vi "Create Spectra Figure 2.0.vi"() -> ()   [LabVIEW 2021]
uses:
  <vilib>/Heliosphere Research LLC/Advanced Plotting Toolkit/api_annotations/LabelProperties.ctl
  <vilib>/Heliosphere Research LLC/Advanced Plotting Toolkit/properties/Text.ctl
  <vilib>/Heliosphere Research LLC/Advanced Plotting Toolkit/typedefs/PlotColor.ctl
  <vilib>/Heliosphere Research LLC/Advanced Plotting Toolkit/properties/Text_FontSize.ctl
  <vilib>/Heliosphere Research LLC/Advanced Plotting Toolkit/properties/Text_FontStyle.ctl
  <vilib>/Heliosphere Research LLC/Advanced Plotting Toolkit/api_figure/TicksProperties.ctl
  <vilib>/Heliosphere Research LLC/Advanced Plotting Toolkit/api_plotting/LineProperties.ctl
  <vilib>/Heliosphere Research LLC/Advanced Plotting Toolkit/properties/Line.ctl
  <vilib>/Heliosphere Research LLC/Advanced Plotting Toolkit/properties/Line_Style.ctl
  <vilib>/Heliosphere Research LLC/Advanced Plotting Toolkit/properties/Marker.ctl
  <vilib>/Heliosphere Research LLC/Advanced Plotting Toolkit/properties/Marker_Style.ctl
  <vilib>/Heliosphere Research LLC/Advanced Plotting Toolkit/properties/Display.ctl
  <vilib>/regexp/Match Regular Expression.xnode
  <vilib>/Heliosphere Research LLC/Advanced Plotting Toolkit/Advanced Plotting Toolkit.lvlib
  <vilib>/Analysis/NI_AALPro.lvlib
panel:
  out "Pressure":picture
  out "Speed Profiles":picture
  out "Full Spectrum":picture
  out "Trimmed Spectra":picture
  out "Bar Plot":picture
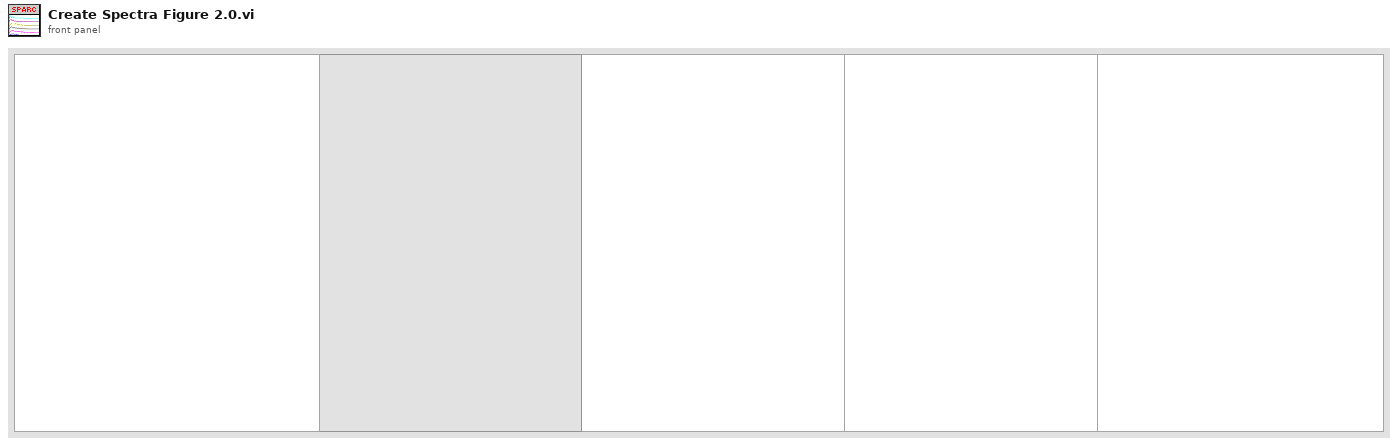
[diagram p1: front panel]
types:
  T1 = typedef "Advanced Plotting Toolkit.lvlib/LineProperties.ctl" = cluster{"Line":T2, "Marker":T5, "Display":T7}
  T2 = typedef "Advanced Plotting Toolkit.lvlib/Line.ctl" = cluster{"Style":T3, "Color":T4, "Width":sgl}
  T3 = typedef "Advanced Plotting Toolkit.lvlib/Line_Style.ctl" = enum16{"Automatic", "Solid", "Dashed", "Dotted", "Dash-dot", "Invisible"}
  T4 = typedef "Advanced Plotting Toolkit.lvlib/PlotColor.ctl" = u32
  T5 = typedef "Advanced Plotting Toolkit.lvlib/Marker.ctl" = cluster{"Style":T6, "Color":T4, "Size":dbl}
  T6 = typedef "Advanced Plotting Toolkit.lvlib/Marker_Style.ctl" = enum16{"Automatic", "Circle", "Square", "Triangle", "Diamond", "Star", "Invisible"}
  T7 = typedef "Advanced Plotting Toolkit.lvlib/Display.ctl" = cluster{"Alpha":dbl, "Z Order":dbl}
  T8 = typedef "Advanced Plotting Toolkit.lvlib/TicksProperties.ctl" = cluster{"Text":T9}
  T9 = typedef "Advanced Plotting Toolkit.lvlib/Text.ctl" = cluster{"Color":T4, "Background Color":T4, "Font Size (points)":T10, "Font Style":T11, "Rotation Angle":dbl}
  T10 = typedef "Advanced Plotting Toolkit.lvlib/Text_FontSize.ctl" = i32
  T11 = typedef "Advanced Plotting Toolkit.lvlib/Text_FontStyle.ctl" = enum16{"Automatic", "Normal", "Italic", "Bold"}
  T12 = typedef "Advanced Plotting Toolkit.lvlib/LabelProperties.ctl" = cluster{"Text":T9}
  T13 = typedef "Advanced Plotting Toolkit.lvlib/PlotID.ctl" = i32
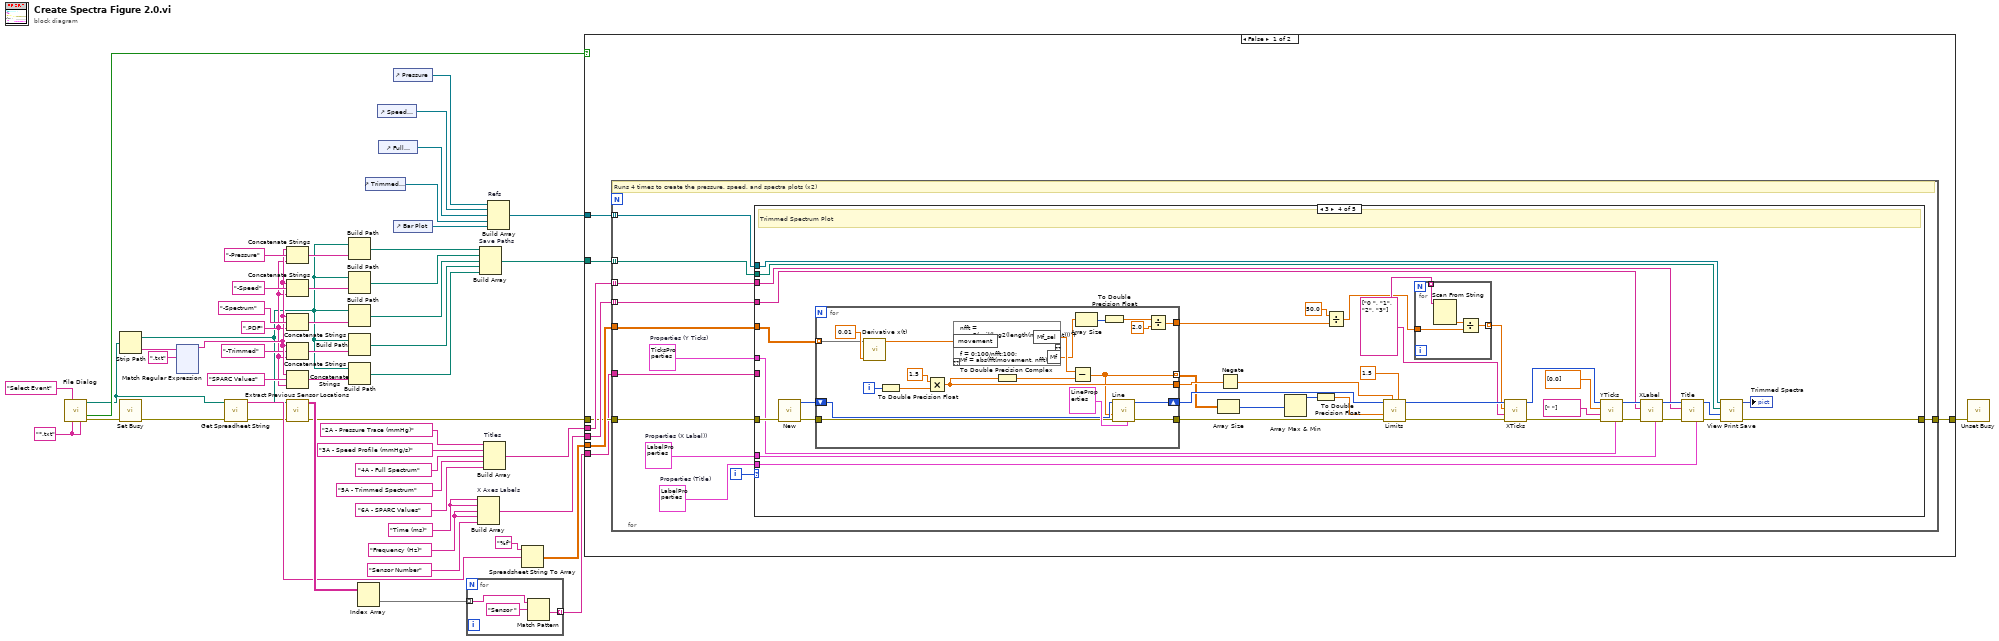
[diagram p0: block diagram]
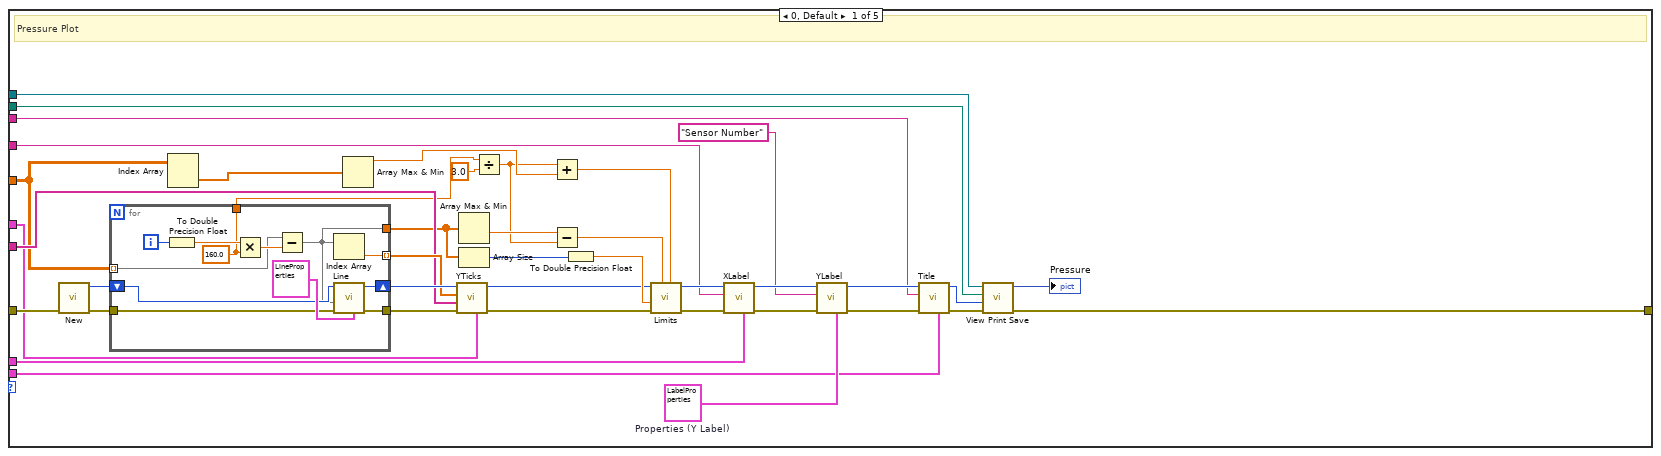
[diagram p2: hidden frame]
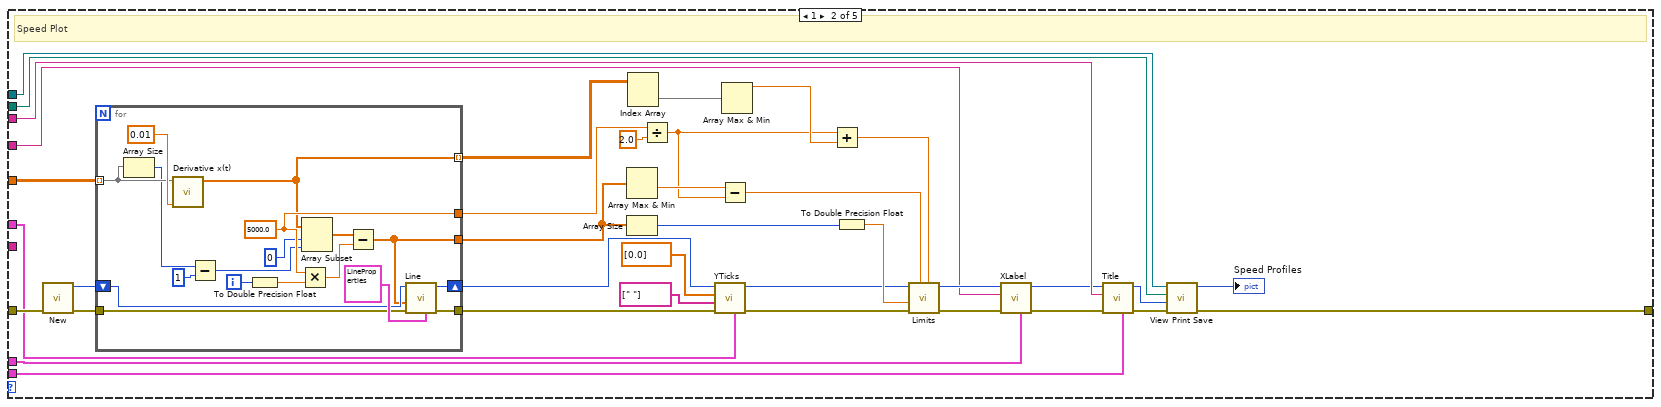
[diagram p3: hidden frame]
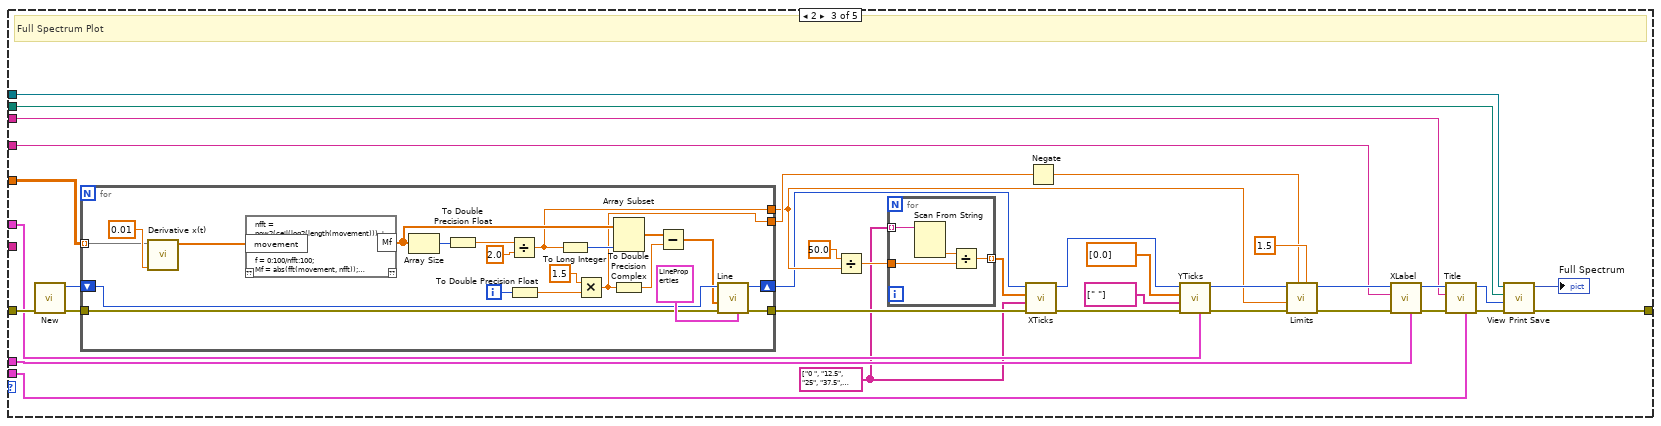
[diagram p4: hidden frame]
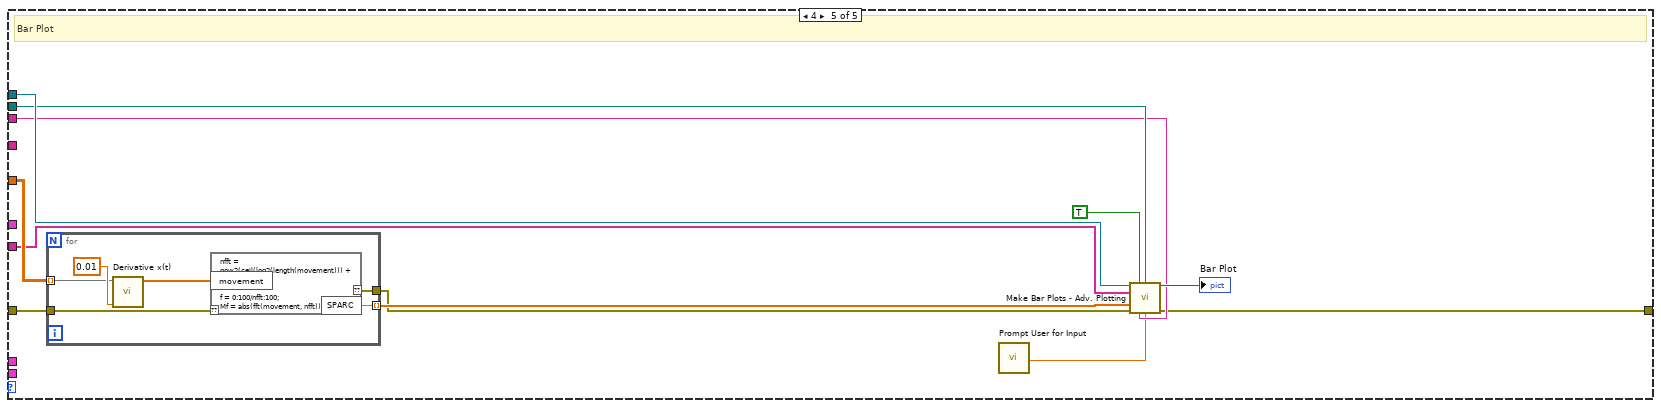
[diagram p5: hidden frame]
diagram:
  w20 = ".PDF" ("string")
  w38 = "Frequency (Hz)" ("Label")
  w39 = "Time (ms)" ("Label")
  w49 = "*.txt" ("pattern label")
  n1 = call "File Dialog"("prompt"="Select Event", "pattern (all files)"=w49, "pattern label"=w49) -> ("selected path"=w26:path, "cancelled"=w51:bool, "error out"=w45:errorcluster)  [unwired: 9 in, 1 out]
  n2 = Strip Path(path=w26) -> (stripped path=w4:path, name=w35:string)
  n3 = call <vilib>:"Set Busy.vi"("error in (no error)"=w45) -> ("error out"=w3:errorcluster)  [unwired: 9 in, 1 out]
  n4 = xnode "Match Regular Expression"("input string"=w35, "regular expression"=".txt") -> ("before match"=w25:string)  [unwired: 4 in, 4 out]
  n5 = call "Get Spreadheet String.vi"("error in (no error)"=w3, "File Path"=w26) -> ("error out"=w2:errorcluster, "Spreadsheet String"=w46:string)  [unwired: 8 in]
  n6 = Concatenate Strings(w25, "-Pressure" ("string"), w20) -> (w37:string)
  n7 = Concatenate Strings(w25, "-Speed" ("string"), w20) -> (w30:string)
  n8 = Concatenate Strings(w25, "-Spectrum" ("string"), w20) -> (w31:string)
  n9 = Concatenate Strings(w25, "-Trimmed" ("string"), w20) -> (w22:string)
  n10 = Concatenate Strings(w25, "SPARC Values" ("string"), w20) -> (w32:string)
  n11 = call "Extract Previous Sensor Locations.vi"("error in (no error)"=w2, "Folder Path"=w4) -> ("error out"=w1:errorcluster, "Sensors"=w47:string[][])  [unwired: 7 in, 1 out]
  n12 = Build Path(base path=w4, name or relative path=w37) -> (appended path=w33:path)
  n13 = Build Path(base path=w4, name or relative path=w30) -> (appended path=w24:path)
  n14 = Build Path(base path=w4, name or relative path=w31) -> (appended path=w23:path)
  n15 = Build Path(base path=w4, name or relative path=w22) -> (appended path=w19:path)
  n16 = Build Path(base path=w4, name or relative path=w32) -> (appended path=w8:path)
  n17 = Index Array(array=w47) -> (element=w44:string[])  [unwired: 2 in]
  n18 = control-ref of="Trimmed Spectra"() -> (w12:refnum<vi>)
  n19 = control-ref of="Speed Profiles"() -> (w14:refnum<vi>)
  n20 = control-ref of="Full Spectrum"() -> (w13:refnum<vi>)
  n21 = control-ref of="Pressure"() -> (w15:refnum<vi>)
  n22 = control-ref of="Bar Plot"() -> (w9:refnum<vi>)
  n23 = for {
    tunnel: w44 -> [w55] mode=indexing
    tunnel: [w53] -> w7 mode=indexing
    n24 = Match Pattern(string=w55, regular expression="Sensor ") -> (after substring=w53:string)  [unwired: 1 in, 3 out]
  }
  n25 = Build Array "X Axes Labels"(w39, w39, w38, w38, "Sensor Number" ("Label")) -> (w16:string[])
  n26 = Build Array "Save Paths"(w33, w24, w23, w19, w8) -> (w17:path[])
  n27 = Build Array "Titles"("2A - Pressure Trace (mmHg)" ("Title"), "3A - Speed Profile (mmHg/s)" ("Title"), "4A - Full Spectrum" ("Title"), "5A - Trimmed Spectrum" ("Title"), "6A - SPARC Values" ("Title")) -> (w18:string[])
  n28 = Build Array "Refs"(w15, w14, w13, w12, w9) -> (w11:refnum<vi>[])
  n29 = Spreadsheet String To Array(format string="%f", spreadsheet string=w46) -> (array=w48:dbl[][])  [unwired: 2 in]
  n30 = case shown="False" w51 {
    tunnel: w1 -> [w58 w324]
    tunnel: w48 -> [w61 _]
    tunnel: w18 -> [w63 _]
    tunnel: w17 -> [w59 _]
    tunnel: w16 -> [w62 _]
    tunnel: w11 -> [w60 _]
    tunnel: [w57 w324] -> w10
    tunnel: w7 -> [w56 _]
    frame False {
      n31 = for {
        tunnel: w63 -> [w69] mode=indexing
        tunnel: w62 -> [w65] mode=indexing
        tunnel: w61 -> [w72]
        tunnel: w60 -> [w73] mode=indexing
        tunnel: w59 -> [w74] mode=indexing
        tunnel: w58 -> [w71]
        tunnel: [w70] -> w57
        tunnel: w56 -> [w68]
        i -> [w75]
        w64 = T8 {"Text"={"Color"=2147483647, "Background Color"=2147483647, "Font Size (points)"=-3, "Font Style"=enum."Bold", "Rotation Angle"=0.0}}  # Properties (Y Ticks)
        w66 = T12 {"Text"={"Color"=2147483647, "Background Color"=2147483647, "Font Size (points)"=-3, "Font Style"=enum."Bold", "Rotation Angle"=nan}}  # Properties (X Label))
        w67 = T12 {"Text"={"Color"=2147483647, "Background Color"=2147483647, "Font Size (points)"=-4, "Font Style"=enum."Bold", "Rotation Angle"=nan}}  # Properties (Title)
        # "Runs 4 times to create the pressure, speed, and spectra plots (x2)"
        n32 = case shown="3" w75 {
          tunnel: w74 -> [w115 w163 w216 w279 w312]
          tunnel: w73 -> [w114 w164 w217 w280 w313]
          tunnel: w72 -> [w81 w148 w196 w276 w315]
          tunnel: w71 -> [w110 w158 w212 w275 w307]
          tunnel: [w109 w161 w211 w274 w309] -> w70
          tunnel: w69 -> [w103 w139 w200 w265 w311]
          tunnel: w68 -> [w88 _ _ _ w310]
          tunnel: w67 -> [w102 w142 w195 w264 _]
          tunnel: w66 -> [w76 w138 w198 w262 _]
          tunnel: w65 -> [w95 w143 w199 w263 _]
          tunnel: w64 -> [w77 w130 w197 w261 _]
          frame 0, Default {
            w106 = T12 {"Text"={"Color"=2147483647, "Background Color"=2147483647, "Font Size (points)"=-3, "Font Style"=enum."Bold", "Rotation Angle"=nan}}  # Properties (Y Label)
            # "Pressure Plot"
            n33 = call <vilib>:"New.vi"("error in (no error)"=w110) -> ("error out"=w112:errorcluster, "Plot ID"=w111:T13)  [unwired: 9 in]
            n34 = for {
              tunnel: w81 -> [w119] mode=indexing
              shift-right: [w126] -> w90
              shift-left: w111 -> [w125]
              tunnel: w112 -> [w124]
              tunnel: [w123] -> w93
              tunnel: [w118] -> w84
              tunnel: [w117] -> w89 mode=indexing
              tunnel: [w116] -> w80
              i -> [w122]
              w116 = 160.0 ("y")
              n35 = To Double Precision Float(number=w122) -> (double precision float=w121:dbl)
              n36 = Multiply(x=w121, y=w116) -> (x*y=w120:dbl)
              n37 = Subtract(x=w119, y=w120) -> (x-y=w118:dbl[])
              n38 = Index Array(array=w118) -> (element=w117:dbl)  [unwired: 1 in]
              n39 = call <vilib>:"Line.vi"("Properties"=T1 {"Line"={"Style"=enum."Automatic", "Color"=2147483647, "Width"=2.0}, "Marker"={"Style"=enum."Automatic", "Color"=2147483647, "Size"=nan}, "Display"={"Alpha"=nan, "Z Order"=nan}}, "error in (no error)"=w124, "Y Data"=w118, "Plot ID"=w125) -> ("error out"=w123:errorcluster, "Plot ID out"=w126:T13)  [unwired: 6 in]
            }
            n40 = Index Array(array=w81) -> (element=w87:dbl[])  [unwired: 2 in]
            n41 = Array Max & Min(array=w87) -> (max value=w86:dbl)  [unwired: 3 out]
            n42 = call <vilib>:"YTicks.vi"("Properties"=w77, "error in (no error)"=w93, "Tick Labels"=w88, "Tick Locations"=w89, "Plot ID"=w90) -> ("error out"=w92:errorcluster, "Plot ID Out"=w91:T13)  [unwired: 5 in]
            n43 = Array Max & Min(array=w84) -> (min value=w83:dbl)  [unwired: 3 out]
            n44 = Array Size(array=w84) -> (size(s)=w97:i32)
            n45 = Divide(x=w80, y=3.0) -> (x/y=w78:dbl)
            n46 = Add(x=w78, y=w86) -> (x+y=w85:dbl)
            n47 = Subtract(x=w83, y=w78) -> (x-y=w82:dbl)
            n48 = To Double Precision Float(number=w97) -> (double precision float=w96:dbl)
            n49 = call <vilib>:"Limits.vi"("Y Max"=w85, "Y Min"=w82, "error in (no error)"=w92, "X Max"=w96, "Plot ID"=w91) -> ("error out"=w100:errorcluster, "Plot ID Out"=w99:T13)  [unwired: 5 in]
            n50 = call <vilib>:"XLabel.vi"("Properties"=w76, "error in (no error)"=w100, "Label"=w95, "Plot ID"=w99) -> ("error out"=w101:errorcluster, "Plot ID out"=w98:T13)  [unwired: 6 in]
            n51 = call <vilib>:"YLabel.vi"("Properties"=w106, "error in (no error)"=w101, "Label"="Sensor Number", "Plot ID"=w98) -> ("error out"=w107:errorcluster, "Plot ID out"=w108:T13)  [unwired: 6 in]
            n52 = call <vilib>:"Title.vi"("Properties"=w102, "error in (no error)"=w107, "Title"=w103, "Plot ID"=w108) -> ("error out"=w104:errorcluster, "Plot ID out"=w105:T13)  [unwired: 6 in]
            n53 = call "View Print Save.vi"("error in (no error)"=w104, "Plot ID in"=w105, "appended path"=w115, "Picture in"=w114) -> ("error out"=w109:errorcluster, "Picture"=→"Pressure":picture)  [unwired: 6 in]
          }
          frame 1 {
            # "Speed Plot"
            n54 = call <vilib>:"New.vi"("error in (no error)"=w158) -> ("error out"=w160:errorcluster, "Plot ID"=w159:T13)  [unwired: 9 in]
            n55 = for {
              tunnel: w148 -> [w171] mode=indexing
              shift-right: [w181] -> w141
              shift-left: w159 -> [w180]
              tunnel: w160 -> [w179]
              tunnel: [w178] -> w145
              tunnel: [w173] -> w146
              tunnel: [w172] -> w134
              tunnel: [w165] -> w129 mode=indexing
              i -> [w176]
              w172 = 5000.0 ("x")
              n56 = Array Size(array=w171) -> (size(s)=w170:i32)
              n57 = call <vilib>:"Derivative x(t).vi"("dt"=0.01, "X"=w171) -> ("dX/dt"=w165:dbl[])  [unwired: 8 in, 1 out]
              n58 = Subtract(x=w170, y=1) -> (x-y=w168:i32)
              n59 = To Double Precision Float(number=w176) -> (double precision float=w175:dbl)
              n60 = Multiply(x=w172, y=w175) -> (x*y=w174:dbl)
              n61 = Array Subset(array=w165, index=0, length=w168) -> (w166:dbl[])
              n62 = Subtract(x=w166, y=w174) -> (x-y=w173:dbl[])
              n63 = call <vilib>:"Line.vi"("Properties"=T1 {"Line"={"Style"=enum."Automatic", "Color"=2147483647, "Width"=2.0}, "Marker"={"Style"=enum."Automatic", "Color"=2147483647, "Size"=nan}, "Display"={"Alpha"=nan, "Z Order"=nan}}, "error in (no error)"=w179, "Y Data"=w173, "Plot ID"=w180) -> ("error out"=w178:errorcluster, "Plot ID out"=w181:T13)  [unwired: 6 in]
            }
            n64 = Array Max & Min(array=w146) -> (min value=w150:dbl)  [unwired: 3 out]
            n65 = Array Size(array=w146) -> (size(s)=w155:i32)
            n66 = Index Array(array=w129) -> (element=w128:dbl[])  [unwired: 2 in]
            n67 = Divide(x=w134, y=2.0) -> (x/y=w135:dbl)
            n68 = call <vilib>:"YTicks.vi"("Properties"=w130, "error in (no error)"=w145, "Tick Labels"=string[] [" "], "Tick Locations"=dbl[] [0.0], "Plot ID"=w141) -> ("error out"=w153:errorcluster, "Plot ID Out"=w152:T13)  [unwired: 5 in]
            n69 = Subtract(x=w150, y=w135) -> (x-y=w149:dbl)
            n70 = Array Max & Min(array=w128) -> (max value=w147:dbl)  [unwired: 3 out]
            n71 = Add(x=w135, y=w147) -> (x+y=w151:dbl)
            n72 = To Double Precision Float(number=w155) -> (double precision float=w154:dbl)
            n73 = call <vilib>:"Limits.vi"("Y Max"=w151, "Y Min"=w149, "error in (no error)"=w153, "X Max"=w154, "Plot ID"=w152) -> ("error out"=w157:errorcluster, "Plot ID Out"=w156:T13)  [unwired: 5 in]
            n74 = call <vilib>:"XLabel.vi"("Properties"=w138, "error in (no error)"=w157, "Label"=w143, "Plot ID"=w156) -> ("error out"=w132:errorcluster, "Plot ID out"=w131:T13)  [unwired: 6 in]
            n75 = call <vilib>:"Title.vi"("Properties"=w142, "error in (no error)"=w132, "Title"=w139, "Plot ID"=w131) -> ("error out"=w144:errorcluster, "Plot ID out"=w140:T13)  [unwired: 6 in]
            n76 = call "View Print Save.vi"("error in (no error)"=w144, "Plot ID in"=w140, "appended path"=w163, "Picture in"=w164) -> ("error out"=w161:errorcluster, "Picture"=→"Speed Profiles":picture)  [unwired: 6 in]
          }
          frame 2 {
            w184 = string[] ["0 ", "12.5", "25", "37.5", "50"] ("Tick Labels")
            # "Full Spectrum Plot"
            n77 = call <vilib>:"New.vi"("error in (no error)"=w212) -> ("error out"=w214:errorcluster, "Plot ID"=w213:T13)  [unwired: 9 in]
            n78 = for {
              tunnel: w196 -> [w235] mode=indexing
              shift-right: [w241] -> w187
              shift-left: w213 -> [w240]
              tunnel: w214 -> [w239]
              tunnel: [w238] -> w186
              tunnel: [w226] -> w191
              tunnel: [w222] -> w193
              i -> [w230]
              n79 = call <vilib>:"Derivative x(t).vi"("dt"=0.01, "X"=w235) -> ("dX/dt"=w236:dbl[])  [unwired: 8 in, 1 out]
              n80 = script code="nfft = pow2(ceil(log2(length(movement))) + 4);\n\nf = 0:100/nfft:100;\nMf = abs(fft(movement, nfft));\nMf = Mf/max(Mf);\n\nfc_inx = find(f<=3);\nf_sel = f(fc_inx);\nMf_sel = Mf(fc_inx);\n\n\ninx = find((Mf_sel>=0.01));\nfc_inx = inx(1):inx(end);\nf_sel = f_sel(fc_inx);\nMf_sel = Mf_sel(fc_inx);\n\nSPARC = -sum(sqrt((diff(f_sel)/f_sel(end)-f_sel(1)).^2+(diff(Mf_sel).^2)));"("movement"=w236) -> ("Mf"=w229:cdb[])  [unwired: 1 in, 1 out]
              n81 = Array Size(array=w229) -> (size(s)=w234:i32)
              n82 = To Double Precision Float(number=w234) -> (double precision float=w233:dbl)
              n83 = Divide(x=w233, y=2.0) -> (x/y=w226:dbl)
              n84 = To Double Precision Float(number=w230) -> (double precision float=w231:dbl)
              n85 = To Long Integer(number=w226) -> (32bit integer=w228:i32)
              n86 = Multiply(x=1.5, y=w231) -> (x*y=w222:dbl)
              n87 = Array Subset(array=w229, length=w228) -> (w223:cdb[])  [unwired: 1 in]
              n88 = To Double Precision Complex(1:w222) -> (0:w227:cdb)
              n89 = Subtract(x=w223, y=w227) -> (x-y=w224:cdb[])
              n90 = call <vilib>:"Line.vi"("Properties"=T1 {"Line"={"Style"=enum."Automatic", "Color"=2147483647, "Width"=2.0}, "Marker"={"Style"=enum."Automatic", "Color"=2147483647, "Size"=nan}, "Display"={"Alpha"=nan, "Z Order"=nan}}, "error in (no error)"=w239, "Y Data"=w224, "Plot ID"=w240) -> ("error out"=w238:errorcluster, "Plot ID out"=w241:T13)  [unwired: 6 in]
            }
            n91 = Divide(x=50.0, y=w191) -> (x/y=w185:dbl)
            n92 = for {
              tunnel: w184 -> [w221] mode=indexing
              tunnel: w185 -> [w219]
              tunnel: [w218] -> w183 mode=indexing
              n93 = Scan From String(input string=w221) -> (output 1=w220:dbl)  [unwired: 4 in, 3 out]
              n94 = Divide(x=w220, y=w219) -> (x/y=w218:dbl)
            }
            n95 = call <vilib>:"XTicks.vi"("error in (no error)"=w186, "Tick Labels"=w184, "Tick Locations"=w183, "Plot ID"=w187) -> ("error out"=w189:errorcluster, "Plot ID Out"=w188:T13)  [unwired: 6 in]
            n96 = Negate(x=w193) -> (-x=w192:dbl)
            n97 = call <vilib>:"YTicks.vi"("Properties"=w197, "error in (no error)"=w189, "Tick Labels"=string[] [" "], "Tick Locations"=dbl[] [0.0], "Plot ID"=w188) -> ("error out"=w208:errorcluster, "Plot ID Out"=w207:T13)  [unwired: 5 in]
            n98 = call <vilib>:"Limits.vi"("Y Max"=1.5, "Y Min"=w192, "error in (no error)"=w208, "X Max"=w191, "Plot ID"=w207) -> ("error out"=w210:errorcluster, "Plot ID Out"=w209:T13)  [unwired: 5 in]
            n99 = call <vilib>:"XLabel.vi"("Properties"=w198, "error in (no error)"=w210, "Label"=w199, "Plot ID"=w209) -> ("error out"=w204:errorcluster, "Plot ID out"=w203:T13)  [unwired: 6 in]
            n100 = call <vilib>:"Title.vi"("Properties"=w195, "error in (no error)"=w204, "Title"=w200, "Plot ID"=w203) -> ("error out"=w202:errorcluster, "Plot ID out"=w201:T13)  [unwired: 6 in]
            n101 = call "View Print Save.vi"("error in (no error)"=w202, "Plot ID in"=w201, "appended path"=w216, "Picture in"=w217) -> ("error out"=w211:errorcluster, "Picture"=→"Full Spectrum":picture)  [unwired: 6 in]
          }
          frame 3 {
            w247 = string[] ["0 ", "1", "2", "3"] ("Tick Labels")
            # "Trimmed Spectrum Plot"
            n102 = call <vilib>:"New.vi"("error in (no error)"=w275) -> ("error out"=w278:errorcluster, "Plot ID"=w277:T13)  [unwired: 9 in]
            n103 = for {
              tunnel: w276 -> [w299] mode=indexing
              shift-right: [w304] -> w260
              shift-left: w277 -> [w303]
              tunnel: w278 -> [w302]
              tunnel: [w301] -> w259
              tunnel: [w292] -> w258
              tunnel: [w291] -> w255 mode=indexing
              tunnel: [w286] -> w246
              i -> [w294]
              n104 = call <vilib>:"Derivative x(t).vi"("dt"=0.01, "X"=w299) -> ("dX/dt"=w298:dbl[])  [unwired: 8 in, 1 out]
              n105 = To Double Precision Float(number=w294) -> (double precision float=w293:dbl)
              n106 = Multiply(x=1.5, y=w293) -> (x*y=w292:dbl)
              n107 = script code="nfft = pow2(ceil(log2(length(movement))) + 4);\n\nf = 0:100/nfft:100;\nMf = abs(fft(movement, nfft));\nMf = Mf/max(Mf);\n\nfc_inx = find(f<=3);\nf_sel = f(fc_inx);\nMf_sel = Mf(fc_inx);\n\n\ninx = find((Mf_sel>=0.01));\nfc_inx = inx(1):inx(end);\nf_sel = f_sel(fc_inx);\nMf_sel = Mf_sel(fc_inx);\n\nSPARC = -sum(sqrt((diff(f_sel)/f_sel(end)-f_sel(1)).^2+(diff(Mf_sel).^2)));"("movement"=w298) -> ("Mf_sel"=w295:cdb[], "Mf"=w287:cdb[])  [unwired: 1 in, 1 out]
              n108 = To Double Precision Complex(1:w292) -> (0:w296:cdb)
              n109 = Subtract(x=w295, y=w296) -> (x-y=w291:cdb[])
              n110 = Array Size(array=w287) -> (size(s)=w290:i32)
              n111 = To Double Precision Float(number=w290) -> (double precision float=w289:dbl)
              n112 = call <vilib>:"Line.vi"("Properties"=T1 {"Line"={"Style"=enum."Automatic", "Color"=2147483647, "Width"=2.0}, "Marker"={"Style"=enum."Automatic", "Color"=2147483647, "Size"=nan}, "Display"={"Alpha"=nan, "Z Order"=nan}}, "error in (no error)"=w302, "Y Data"=w291, "Plot ID"=w303) -> ("error out"=w301:errorcluster, "Plot ID out"=w304:T13)  [unwired: 6 in]
              n113 = Divide(x=w289, y=2.0) -> (x/y=w286:dbl)
            }
            n114 = Array Size(array=w255) -> (size(s)=w254:i32[])
            n115 = Negate(x=w258) -> (-x=w257:dbl)
            n116 = Array Max & Min(array=w254) -> (max value=w253:i32)  [unwired: 3 out]
            n117 = To Double Precision Float(number=w253) -> (double precision float=w248:dbl)
            n118 = Divide(x=50.0, y=w246) -> (x/y=w245:dbl)
            n119 = call <vilib>:"Limits.vi"("Y Max"=1.5, "Y Min"=w257, "error in (no error)"=w259, "X Max"=w248, "Plot ID"=w260) -> ("error out"=w249:errorcluster, "Plot ID Out"=w252:T13)  [unwired: 5 in]
            n120 = for {
              tunnel: [w284] -> w243 mode=indexing
              tunnel: w247 -> [w283] mode=indexing
              tunnel: w245 -> [w282]
              n121 = Scan From String(input string=w283) -> (output 1=w285:dbl)  [unwired: 4 in, 3 out]
              n122 = Divide(x=w285, y=w282) -> (x/y=w284:dbl)
            }
            n123 = call <vilib>:"XTicks.vi"("error in (no error)"=w249, "Tick Labels"=w247, "Tick Locations"=w243, "Plot ID"=w252) -> ("error out"=w250:errorcluster, "Plot ID Out"=w251:T13)  [unwired: 6 in]
            n124 = call <vilib>:"YTicks.vi"("Properties"=w261, "error in (no error)"=w250, "Tick Labels"=string[] [" "], "Tick Locations"=dbl[] [0.0], "Plot ID"=w251) -> ("error out"=w272:errorcluster, "Plot ID Out"=w271:T13)  [unwired: 5 in]
            n125 = call <vilib>:"XLabel.vi"("Properties"=w262, "error in (no error)"=w272, "Label"=w263, "Plot ID"=w271) -> ("error out"=w270:errorcluster, "Plot ID out"=w269:T13)  [unwired: 6 in]
            n126 = call <vilib>:"Title.vi"("Properties"=w264, "error in (no error)"=w270, "Title"=w265, "Plot ID"=w269) -> ("error out"=w266:errorcluster, "Plot ID out"=w267:T13)  [unwired: 6 in]
            n127 = call "View Print Save.vi"("error in (no error)"=w266, "Plot ID in"=w267, "appended path"=w279, "Picture in"=w280) -> ("error out"=w274:errorcluster, "Picture"=→"Trimmed Spectra":picture)  [unwired: 6 in]
          }
          frame 4 {
            # "Bar Plot"
            n128 = for {
              tunnel: w315 -> [w322] mode=indexing
              tunnel: [w320] -> w314 mode=indexing
              tunnel: [w319] -> w308
              tunnel: w307 -> [w318]
              n129 = call <vilib>:"Derivative x(t).vi"("dt"=0.01, "X"=w322) -> ("dX/dt"=w321:dbl[])  [unwired: 8 in, 1 out]
              n130 = script code="nfft = pow2(ceil(log2(length(movement))) + 4);\n\nf = 0:100/nfft:100;\nMf = abs(fft(movement, nfft));\nMf = Mf/max(Mf);\n\nfc_inx = find(f<=3);\nf_sel = f(fc_inx);\nMf_sel = Mf(fc_inx);\n\n\ninx = find((Mf_sel>=0.01));\nfc_inx = inx(1):inx(end);\nf_sel = f_sel(fc_inx);\nMf_sel = Mf_sel(fc_inx);\n\nSPARC = -sum(sqrt((diff(f_sel)/f_sel(end)-f_sel(1)).^2+(diff(Mf_sel).^2)));"("??"=w318, "movement"=w321) -> ("??"=w319:errorcluster, "SPARC"=w320:dbl)
            }
            n131 = call "Prompt User for Input"() -> ("Lower Bound"=w306:dbl)  [unwired: 17 in, 2 out]
            n132 = call "Make Bar Plots - Adv. Plotting.vi"("Picture in"=w313, "Save Plot?"=TRUE, "Save Path"=w312, "Labels"=w310, "SPARC"=w314, "error in (no error)"=w308, "Title"=w311, "Y Min"=w306) -> ("Picture"=→"Bar Plot":picture, "error out"=w309:errorcluster)  [unwired: 6 in]
          }
        }
      }
    }
    frame True {
    }
  }
  n133 = call <vilib>:"Unset Busy.vi"("error in (no error)"=w10) -> ()  [unwired: 10 in, 1 out]
